vi "Turret In Range.vi"(0 "Current Angle":dbl) -> (1 "In Range?":bool, 2 "New Angle":dbl)   [LabVIEW 2019]
panel:
  in  "Slide":dbl(slide) scale=-720.0..720.0
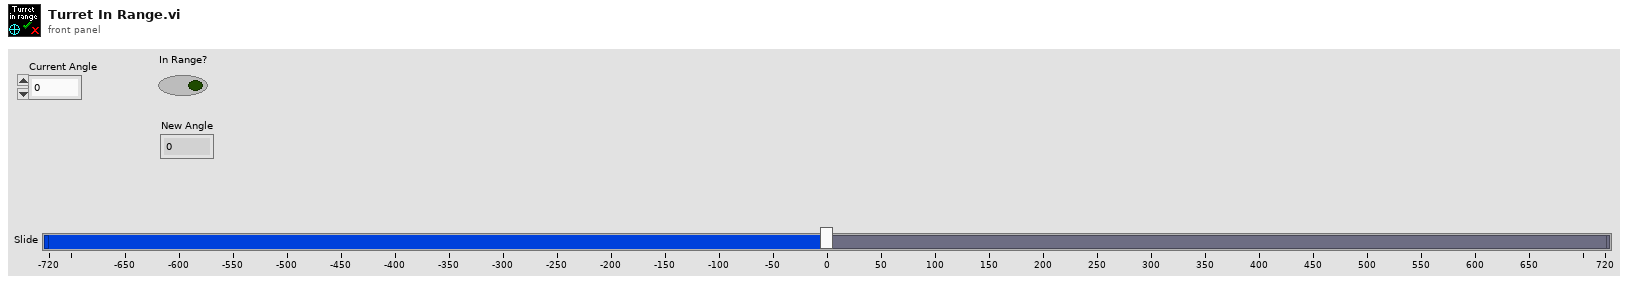
[diagram p1: front panel]
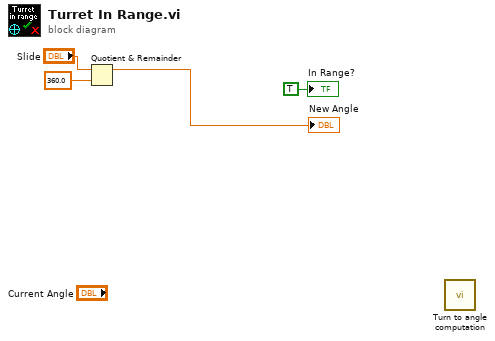
[diagram p0: block diagram]
diagram:
  n1 = Quotient & Remainder(x="Slide", y=360.0) -> (x-y*floor(x/y)=→"New Angle":dbl)  [unwired: 1 out]
  n2 = call "Turn to angle computation.vi"() -> ()  [unwired: 11 in, 1 out]
  "In Range?" <- TRUE ("In Range?")
